vi "Highlight Bottom Entry.vi"(8 "Array.Stats":string[][](array[string]), 9 "Array.Data":string[][](array[string]), 10 "Reference Stats":refnum<vi>, 11 "Reference Data":refnum<vi>) -> ()   [LabVIEW 2013]
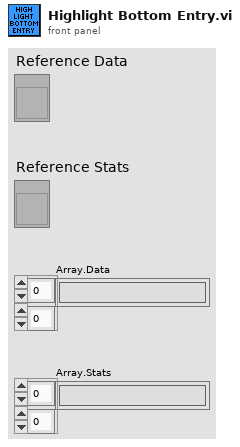
[diagram p1: front panel]
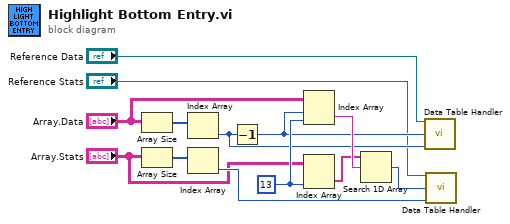
[diagram p0: block diagram]
diagram:
  w10 = 13 ("disabled index (col)")
  n1 = Array Size(array="Array.Data") -> (size(s)=w5:i32[])
  n2 = Array Size(array="Array.Stats") -> (size(s)=w6:i32[])
  n3 = Index Array(array=w5) -> (element=w8:i32)  [unwired: 1 in]
  n4 = Index Array(array=w6) -> (element=w9:i32)  [unwired: 1 in]
  n5 = Decrement(x=w8) -> (x-1=w7:i32)
  n6 = Index Array(array="Array.Data", index (row)=w7, index (col)=w10) -> (element=w12:string)
  n7 = Index Array(array="Array.Stats", index (col)=w10) -> (element=w11:string[])  [unwired: 1 in]
  n8 = Search 1D Array(1D array=w11, element=w12) -> (index of element=w13:i32)  [unwired: 1 in]
  n9 = call "Data Table Handler.vi"("TableRef"="Reference Data", "DesiredRow"=w7, "TableRows"=w8) -> ()  [unwired: 12 in, 1 out]
  n10 = call "Data Table Handler.vi"("TableRef"="Reference Stats", "DesiredRow"=w13, "TableRows"=w9) -> ()  [unwired: 12 in, 1 out]
